vi "Test Find Runs.vi"() -> ()   [LabVIEW 2015]
panel:
  in  "Min Run Length":i32
  out "Length":i32[](array[numeric])
  out "Start":i32[](array[numeric])
  in  "Array":bool[](array[boolean])
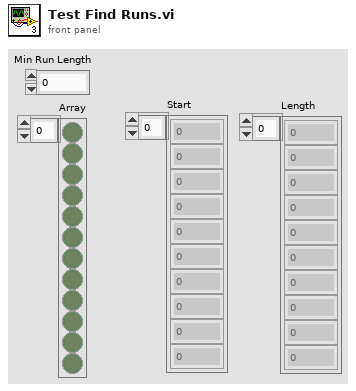
[diagram p1: front panel]
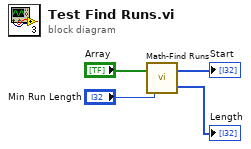
[diagram p0: block diagram]
diagram:
  n1 = call "Math-Find Runs.vi"("Min Run Length"="Min Run Length", "Array"="Array") -> ("Length"=→"Length":i32[], "Start"=→"Start":i32[])
